vi "TrajClosePtAve.vi"(7 "TrajLength":i32, 8 "Dmin_Ave":dbl, 9 "ClosePtIdx_Ave":i32, 10 "Dmin_Target":dbl format="%#.6f", 11 "ClosePtIdx_Target":i32) -> (1 "weightTarget":dbl format="%#.4f", 3 "ClosePtIdx_Ave":i32)   [LabVIEW 2016, in "ForceField.lvclass"]
uses:
  ForceField.lvclass
panel:
  out "Waveform Chart":i32(graph)
  in  "Bias":dbl=0.05
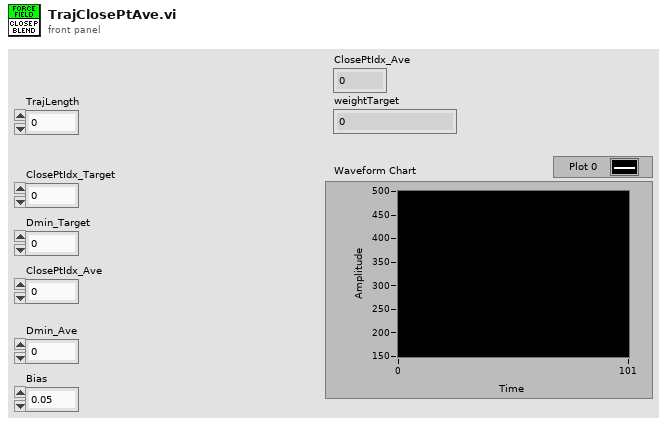
[diagram p1: front panel]
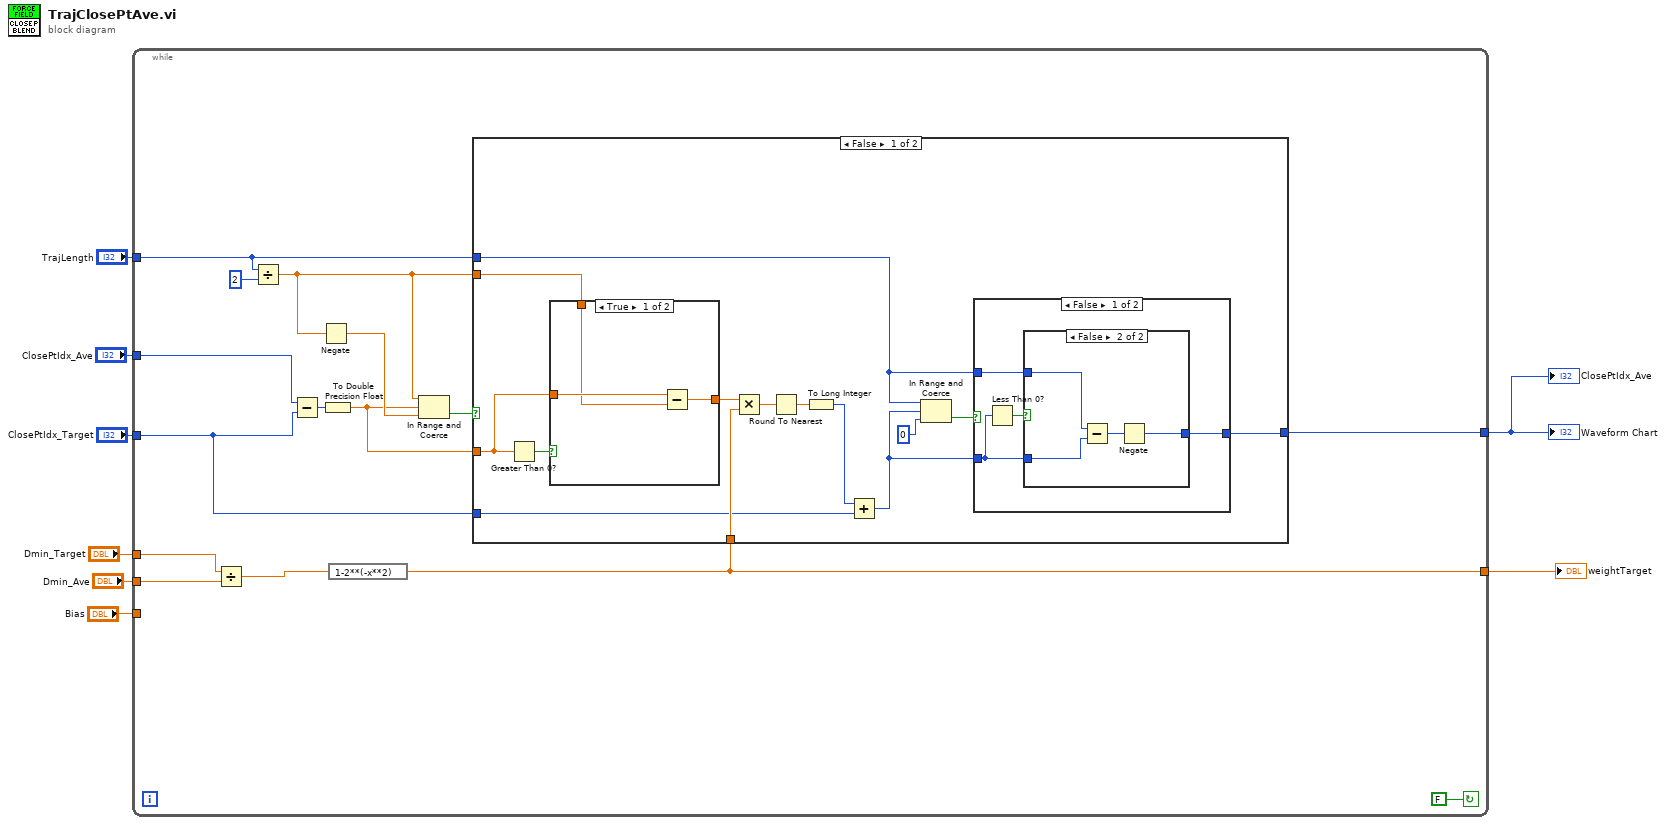
[diagram p0: block diagram]
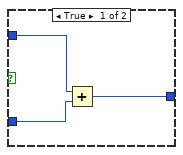
[diagram p2: hidden frame]
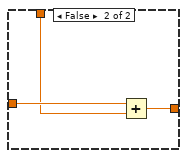
[diagram p4: hidden frame]
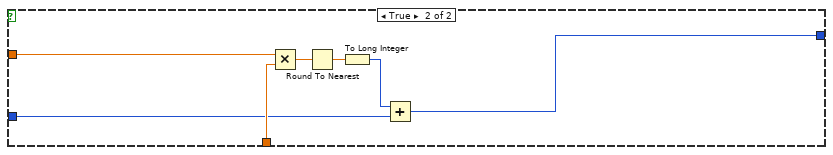
[diagram p5: hidden frame]
diagram:
  n1 = while {
    tunnel: "Bias" -> [_]
    tunnel: "Dmin_Target" -> [w12]
    tunnel: "ClosePtIdx_Ave" -> [w23]
    tunnel: "ClosePtIdx_Target" -> [w16]
    tunnel: "TrajLength" -> [w15]
    tunnel: [w9] -> w3
    tunnel: [w13] -> w2
    tunnel: "Dmin_Ave" -> [w11]
    stop <- FALSE continue-if-true
    n2 = Divide(x=w12, y=w11) -> (x/y=w10:dbl)
    n3 = Divide(x=w15, y=2) -> (x/y=w17:dbl)
    n4 = Subtract(x=w23, y=w16) -> (x-y=w21:i32)
    n5 = Negate(x=w17) -> (-x=w20:dbl)
    n6 = To Double Precision Float(number=w21) -> (double precision float=w18:dbl)
    n7 = expression code="1-2**(-x**2)"(w10) -> (w9:dbl)
    n8 = In Range and Coerce(upper limit=w17, x=w18, lower limit=w20) -> (In Range?=w19:bool)  [unwired: 1 out]
    n9 = case shown="False" w19 {
      tunnel: w9 -> [w33 w62]
      tunnel: w18 -> [w35 w57]
      tunnel: w17 -> [w36 _]
      tunnel: w16 -> [w32 w61]
      tunnel: w15 -> [w25 _]
      tunnel: [w24 w56] -> w13
      frame False {
        n10 = Greater Than 0?(x=w35) -> (x > 0?=w37:bool)
        n11 = case shown="True" w37 {
          tunnel: w36 -> [w51 w54]
          tunnel: w35 -> [w52 w55]
          tunnel: [w50 w53] -> w34
          frame True {
            n12 = Subtract(x=w52, y=w51) -> (x-y=w50:dbl)
          }
          frame False {
            n13 = Add(x=w55, y=w54) -> (x+y=w53:dbl)
          }
        }
        n14 = Multiply(x=w34, y=w33) -> (x*y=w31:dbl)
        n15 = Round To Nearest(number=w31) -> (nearest integer value=w30:dbl)
        n16 = To Long Integer(number=w30) -> (32bit integer=w29:i32)
        n17 = Add(x=w29, y=w32) -> (x+y=w26:i32)
        n18 = In Range and Coerce(upper limit=w25, x=w26, lower limit=0) -> (In Range?=w27:bool)  [unwired: 1 out]
        n19 = case shown="False" w27 {
          tunnel: w26 -> [w40 w49]
          tunnel: w25 -> [w39 _]
          tunnel: [w38 w49] -> w24
          frame False {
            n20 = Less Than 0?(x=w40) -> (x < 0?=w41:bool)
            n21 = case shown="False" w41 {
              tunnel: w40 -> [w44 w48]
              tunnel: w39 -> [w43 w47]
              tunnel: [w42 w45] -> w38
              frame True {
                n22 = Add(x=w43, y=w44) -> (x+y=w42:i32)
              }
              frame False {
                n23 = Subtract(x=w47, y=w48) -> (x-y=w46:i32)
                n24 = Negate(x=w46) -> (-x=w45:i32)
              }
            }
          }
          frame True {
          }
        }
      }
      frame True {
        n25 = Multiply(x=w57, y=w62) -> (x*y=w60:dbl)
        n26 = Round To Nearest(number=w60) -> (nearest integer value=w59:dbl)
        n27 = To Long Integer(number=w59) -> (32bit integer=w58:i32)
        n28 = Add(x=w58, y=w61) -> (x+y=w56:i32)
      }
    }
  }
  "ClosePtIdx_Ave" <- w2
  "weightTarget" <- w3
  "Waveform Chart" <- w2
